vi "getSize.vi"(8 "error in (no error)":errorcluster, 11 "HashMap in":refnum<class "HashMap.lvclass">) -> (0 "error out":errorcluster, 2 "Size":u32, 3 "HashMap out":refnum<class "HashMap.lvclass">)   [LabVIEW 2017, in "HashMap.lvclass"]
uses:
  <userlib>/836-Library/Data_Structures/HashMap/HashMap.lvclass
  <userlib>/836-Library/Data_Structures/HashMap/HashMap.lvclass/HashMap.ctl
  <userlib>/836-Library/Data_Structures/Bucket/Bucket.lvclass
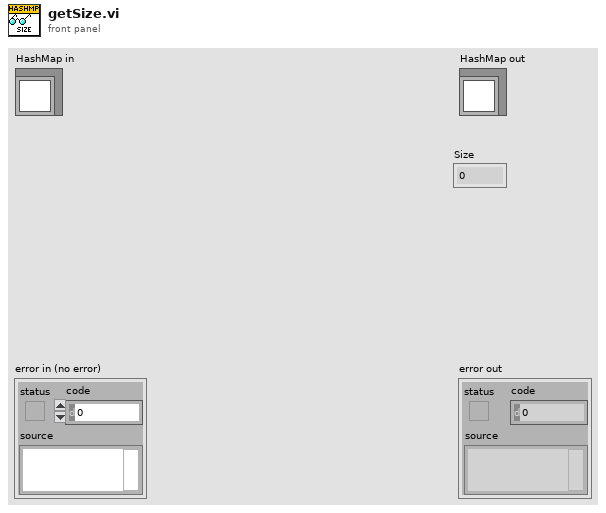
[diagram p1: front panel]
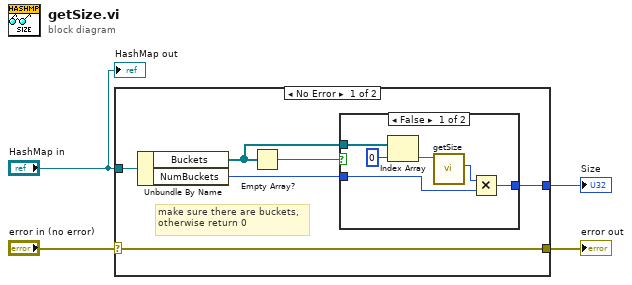
[diagram p0: block diagram]
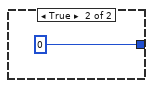
[diagram p2: hidden frame]
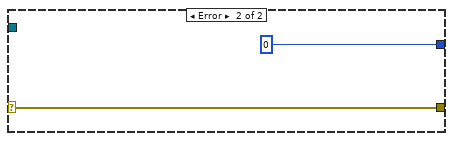
[diagram p3: hidden frame]
diagram:
  n1 = case shown="No Error" "error in (no error)" {
    selector: "error in (no error)" -> [w10 w19]
    tunnel: [w10 w19] -> w3
    tunnel: "HashMap in" -> [w9 _]
    tunnel: [w5 u32 0] -> w1
    frame No Error {
      # "make sure there are buckets,\notherwise return 0"
      n2 = Unbundle By Name(w9) -> ("Buckets"=w6:refnum<class "Bucket.lvclass">[], "NumBuckets"=w8:u32)
      n3 = Empty Array?(array=w6) -> (empty?=w7:bool)
      n4 = case shown="False" w7 {
        tunnel: w8 -> [w13 _]
        tunnel: w6 -> [w12 _]
        tunnel: [w11 u32 0] -> w5
        frame False {
          n5 = Index Array(array=w12, index=0) -> (element=w15:refnum<class "Bucket.lvclass">)
          n6 = call <userlib>:"getSize.vi"("Bucket in"=w15) -> ("Size"=w14:u32)  [unwired: 8 in, 2 out]
          n7 = Multiply(x=w14, y=w13) -> (x*y=w11:u32)
        }
        frame True {
        }
      }
    }
    frame Error {
    }
  }
  "error out" <- w3
  "Size" <- w1
  "HashMap out" <- "HashMap in"
